vi "#SubVI_Sin.vi"(11 "Freq":dbl=1.0) -> (3 "Waveform Graph":dbl[](graph))   [LabVIEW 2019]
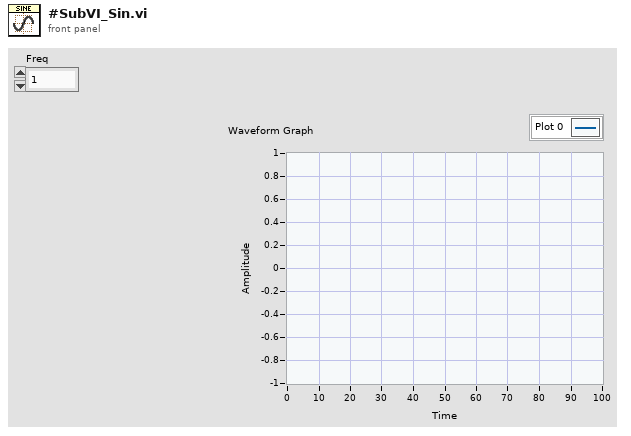
[diagram p1: front panel]
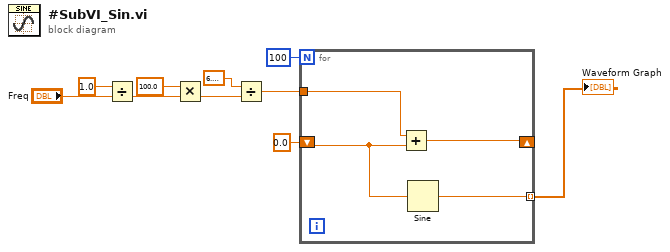
[diagram p0: block diagram]
diagram:
  n1 = Divide(x=1.0, y="Freq") -> (x/y=w4:dbl)
  n2 = Multiply(x=100.0, y=w4) -> (x*y=w6:dbl)
  n3 = Divide(x=6.283185307179586, y=w6) -> (x/y=w8:dbl)
  n4 = for {
    N: 100 -> [_]
    shift-right: [w14] -> _
    shift-left: 0.0 -> [w12]
    tunnel: w8 -> [w13]
    tunnel: [w11] -> w7 mode=indexing
    n5 = Add(x=w13, y=w12) -> (x+y=w14:dbl)
    n6 = Sine(x=w12) -> (sin(x)=w11:dbl)
  }
  "Waveform Graph" <- w7
